vi "LAGetHistory.vi"(8 "Error Input":errorcluster, 11 "LiteAgent In":T1) -> (0 "Error Output":errorcluster, 2 "HistoryJson":string, 3 "LiteAgent Out":T1)   [LabVIEW 2017, in "LiteAgentSDK.lvlib"]
uses:
  LiteAgentSDK.lvlib
  C:/Users/Jan/Projects/LiteAgentSDK-LabVIEW/Source/Bin/LiteAgentSDK.LabVIEW.dll
  Bin/LiteAgentSDK.LabVIEW.dll
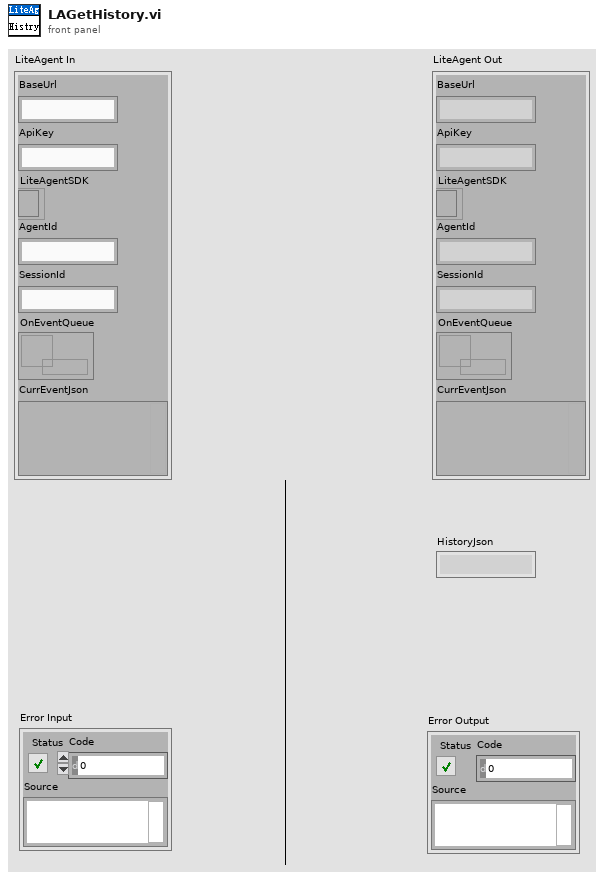
[diagram p1: front panel]
types:
  T1 = cluster{"BaseUrl":string, "ApiKey":string, "LiteAgentSDK":refnum<k24>, "AgentId":string, "SessionId":string, "OnEventQueue":refnum<queue>, "CurrEventJson":variant}
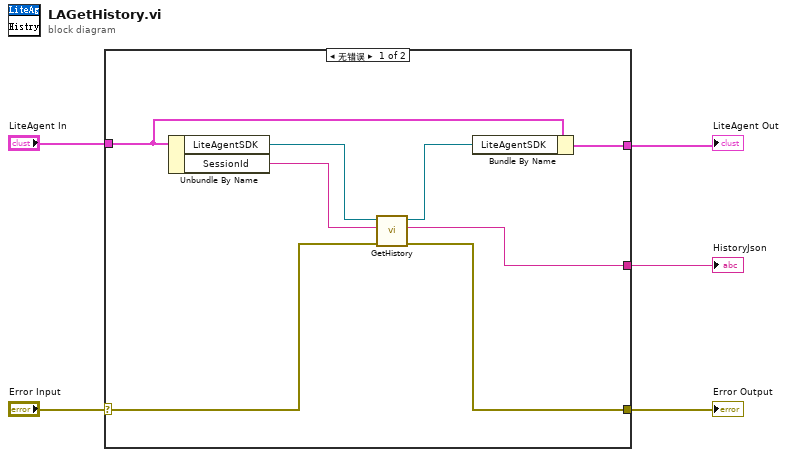
[diagram p0: block diagram]
diagram:
  n1 = case shown="无错误" "Error Input" {
    selector: "Error Input" -> [w13 w15]
    tunnel: [w12 w15] -> w4
    tunnel: [w11 _] -> w3
    tunnel: "LiteAgent In" -> [w10 w14]
    tunnel: [w9 w14] -> w1
    frame No Error {
      n2 = Unbundle By Name(w10) -> ("LiteAgentSDK"=w8:refnum<k24>, "SessionId"=w6:string)
      n3 = call "GetHistory.vi"("Error Input"=w13, "SessionId"=w6, "LiteAgentSDK Input"=w8) -> ("Error Output"=w12:errorcluster, "HistoryJson"=w11:string, "LiteAgentSDK Output"=w7:refnum<k24>)  [unwired: 6 in]
      n4 = Bundle By Name(cluster=w10, "LiteAgentSDK"=w7) -> (w9:T1)
    }
    frame Error {
    }
  }
  "Error Output" <- w4
  "HistoryJson" <- w3
  "LiteAgent Out" <- w1
